vi "事件结构+定时循环模式.vi"() -> ()   [LabVIEW 2013]
uses:
  <vilib>/Platform/TimedLoop/XDataNode/timing_clust.ctl
  <vilib>/Platform/TimedLoop/XDataNode/nitl_modes.ctl
  <vilib>/Platform/TimedLoop/XDataNode/wakeup.ctl
  <vilib>/Platform/TimedLoop/XDataNode/XDataNode.xnode
  <vilib>/Platform/TimedLoop/XDataNode/XDNodeRunTimeDep.lvlib
panel:
  out "采集温度":dbl
  out "采集速度":dbl
  in  "停止":bool
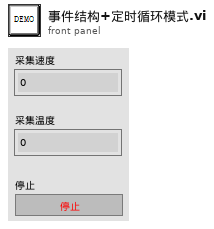
[diagram p1: front panel]
types:
  T1 = typedef "XDNodeRunTimeDep.lvlib/timing_clust.ctl" = cluster{"Expected End [f-1]":u64, "Actual End [f-1]":u64, "Finished Late? [f-1]":bool, "Expected End [i-1]":u64, "Actual End [i-1]":u64, "Finished Late? [i-1]":bool, "Expected Start [i]":u64, "Actual Start [i]":u64, "Expected Start [f]":u64, "Actual Start [f]":u64, "Source Name":string, "Structure Name":string, "Period":i64, "Deadline":i64, "Offset":i64, "Start":i64, "Priority":i32, "Timeout":i32, "Mode":T2, "Wakeup Reason":T3, "Error":errorcluster, "Source Type":string, "Secondary Source Type":string, "Global End Time":u64, "Global Start Time":u64, "Frame Duration":u64, "Iteration Duration":u64, "Assigned CPU":i32, "I/O Scan Engine Mode":u32}
  T2 = typedef "XDNodeRunTimeDep.lvlib/nitl_modes.ctl" = enum32{"No Change", "Process missed periods, maintain original phase", "Discard missed periods, maintain original phase", "Process missed periods, ignore original phase", "Discard missed periods, ignore original phase"}
  T3 = typedef "XDNodeRunTimeDep.lvlib/wakeup.ctl" = enum32{"Normal", "Aborted", "Asynchronous wakeup", "Timing source error", "Timed loop error", "Timeout"}
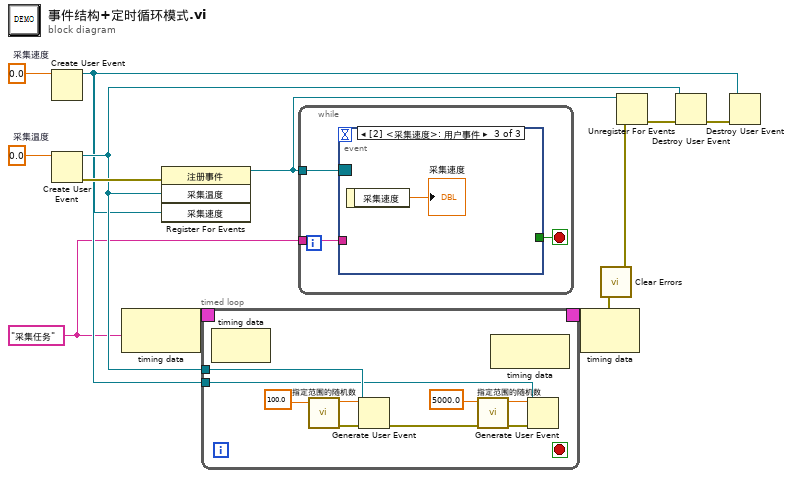
[diagram p0: block diagram]
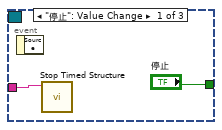
[diagram p2: hidden frame]
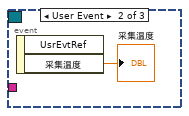
[diagram p3: hidden frame]
diagram:
  w3 = "采集任务" ("结构名称")
  w11 = 0.0  # 采集速度
  w13 = 0.0  # 采集温度
  n1 = Create User Event(user event datatype=w11) -> (user event=w4:refnum<user-event>)  [unwired: 1 in, 1 out]
  n2 = Create User Event(user event datatype=w13) -> (user event=w6:refnum<user-event>, error out=w12:errorcluster)  [unwired: 1 in]
  n3 = node-c288(w3) -> (w10:T1)
  n4 = register-events(error in=w12, w6, w4) -> (reference out=w7:refnum<event-registration>)  [unwired: 1 in, 1 out]
  n5 = timed-loop {
    timing: w10 -> [_]
    timing-out: [_] -> w9
    tunnel: w6 -> [w20]
    tunnel: w4 -> [w15]
    stop <- _ stop-if-true
    n6 = node-c288() -> ()  [unwired: 1 in, 1 out]
    n7 = call-poly "指定范围的随机数.vi"("上限 (1.00)"=100.0) -> ("Error Out"=w18:errorcluster, "随机数"=w19:dbl)  [unwired: 9 in]
    n8 = Generate User Event(user event=w20, event data cluster=w19, error in=w18) -> (error out=w17:errorcluster)  [unwired: 1 in, 1 out]
    n9 = call-poly "指定范围的随机数.vi"("上限 (1.00)"=5000.0, "Error In"=w17) -> ("Error Out"=w16:errorcluster, "随机数"=w14:dbl)  [unwired: 8 in]
    n10 = node-c288() -> ()  [unwired: 1 in, 1 out]
    n11 = Generate User Event(user event=w15, event data cluster=w14, error in=w16) -> ()  [unwired: 1 in, 2 out]
  }
  n12 = while {
    tunnel: w7 -> [w26]
    tunnel: w3 -> [w25]
    stop <- w27 stop-if-true
    n13 = event shown="[2] <采集速度>: 用户事件" {
      selector: w26 -> [_ _ _]
      dyn-events: _ -> [_ _ _]
      timeout: _ -> [_ _ _]
      tunnel: ["停止" _ _] -> w27
      tunnel: w25 -> [w28 _ _]
      event "停止": Value Change {
        n14 = event-data() -> ()  [unwired: 1 in, 1 out]
        n15 = call <vilib>:"Stop Timed Structure.vi"("name"=w28) -> ()  [unwired: 10 in, 1 out]
      }
      event User Event {
        n16 = event-data() -> ("采集温度"=→"采集温度":dbl)  [unwired: 1 in, 1 out]
      }
      event User Event {
        n17 = event-data() -> ("采集速度"=→"采集速度":dbl)  [unwired: 1 in]
      }
    }
  }
  n18 = node-c288(w9) -> (w2:errorcluster)
  n19 = call <vilib>:"Clear Errors.vi"("error in (no error)"=w2) -> ("error out"=w1:errorcluster)  [unwired: 6 in]
  n20 = Unregister For Events(event registration refnum=w7, error in=w1) -> (error out=w8:errorcluster)
  n21 = Destroy User Event(user event=w6, error in=w8) -> (error out=w5:errorcluster)
  n22 = Destroy User Event(user event=w4, error in=w5) -> ()  [unwired: 1 out]
